vi "Untitled 4.vi"() -> ()   [LabVIEW 2011]
uses:
  emi Lib/System 01/0 - General/App/Loop control 2/Private/_emi_SMLoop Control Single.vi
  emi Lib/System 01/0 - General/S&E reporting/Private/_emi_ S&E Message type.ctl
  emi Lib/System 01/0 - General/S&E reporting/Private/_emi_ S&E Message.ctl
  <vilib>/Utility/file.llb/Write To Spreadsheet File (I64).vi
  emi Lib/System 01/0 - General/App/Loop control 2/Private/_emi_SMLoop Get State Single.vi
  Defenitions/LEIN Structure variations.ctl
  Defenitions/Error_system_def.ctl
  Defenitions/err/Controller error.ctl
  Defenitions/LEIN STAT 14 Debug system cluster.ctl
  Nodes/Controller local stat2.ctl
  Nodes/pressure stat2.ctl
  Nodes/solonoid stat2.ctl
  Tool/Stroker/Stat def/Stroker system stat2.ctl
  Defenitions/LEIN CMD List.ctl
  Defenitions/LEIN CMD Cluster.ctl
  Defenitions/LEIN cycle holder.ctl
  Defenitions/LEIN Reply Holder.ctl
  Defenitions/LEIN custom reply Q.ctl
  Nodes/tensionsub stat2.ctl
  Nodes/PSU stat2.ctl
  emi Lib/System 01/0 - General/App/Loop control/Private/_emi Loop status.ctl
  Defenitions/stat2/system status/Stat2 system task info.ctl
panel:
  out "Controller local.relay_status":u8 format="%.0b"
  out "controller task":T1
  out "pressure 2":bool
  out "Pressure 1":bool
  out "Solonoid":bool
  out "pressure 2":T2 {"sys register" format="%04x"}
  out "pressure 1":T2 {"sys register" format="%04x"}
  out "Solonoid":T1
  out "solonoid":T3 {"valve status" format="%02x"; "sys register" format="%04x"}
  out "Error":T4 {"system def error"."Module error mask" format="%08b"}
  out "Debug":T6
  out "ID":T7 {"LEIN implementation" format="%.0x"}
  out "Controler ID":u8[](array[numeric]) format="%.0x"
  out "Controler Debug":u8[](array[numeric]) format="%.0x"
  out "Controler error codes":u8[](array[numeric]) format="%.0x"
  in  "GetID Codes":bool
  in  "Get Debug codes":bool
  in  "Gett erro codes":bool
  out "DATA 3":u8[](array[numeric]) format="%.0x"
  in  "Array 2":u8[](array[numeric])=[1, 0, 1, 1, 2]
  in  "Solonoid":bool
  in  "Restart node":bool
  in  "TASK Data":u8[](array[numeric])=[120, 0, 50, 0, 0]
  in  "TASK ID":u8=49 format="%.0x"
  in  "TASK":bool
  in  "Reset err":bool
  out "DATA 2":u8[](array[numeric])=[240, 3, 105, 1, 0, 243, 11, 2, 32, 0, 6] format="%.0x"
  out "Reply":T8={"SID"=0, "ANF"=FALSE, "CMD"=enum."TASK", "DATA"=[]}
  in  "STAT ID":u8
  out "Numeric":i32
  out "PAss through answer":T8={"SID"=0, "ANF"=FALSE, "CMD"=enum."TASK", "DATA"=[]}
  out "SID 2":u8
  in  "Enable STAT2":bool=TRUE
  in  "Pass through":bool
  out "Boolean":bool
  in  "Ping":bool
  out "CMD":T8={"SID"=0, "ANF"=FALSE, "CMD"=enum."TASK", "DATA"=[]}
  in  "Stat":bool
  in  "Expected LEN":u16=60
  out "tid":u32
  out "PC-Control com errors":u32(graph)
  out "Node connected":u32(graph)
  out "Controller  current":u32(graph)
  out "Node  OSC":u32(graph)
  out "Node transducer":u32(graph)
  out "Node Temperature":u32(graph)
  out "Controller voltage":u32(graph)
  out "Accelerometer Ch 5":u32(graph)
  out "Accelerometer Ch 4":u32(graph)
  out "Accelerometer Ch 3":u32(graph)
  out "Accelerometer Ch 2":u32(graph)
  out "Accelerometer Ch 1":u32(graph)
  out "Accelerometer Ch 0":u32(graph)
  out "Sensor 2":u32(graph)
  out "Sensor 1":u32(graph)
  out "Temperature":u32(graph)
  out "Array":errorcluster[](array[cluster])
  in  "VISA com no":refnum<visa-resource-name>="COM 7"
  out "Loops":T10[](array[typedef])
  out "Received":i32
  out "Transmitt Qd":i32
  out "DATA":u8[](array[numeric]) format="%.0x"
  in  "SID":u8=42
  out "LEIN received":T8={"SID"=0, "ANF"=FALSE, "CMD"=enum."TASK", "DATA"=[]}
  # "In file: Tid, temperature, sensor 1,sensor 2,Acc 0, Acc1, Acc2, Acc3, Acc4, Acc5, Voltage, Current, Com errors, Node temperature, node transducerm, node osc, node discon (0 = connected)"
  # "OBS 1.2 diff OSCTUN location then 1.1"
  # "STAT DATA"
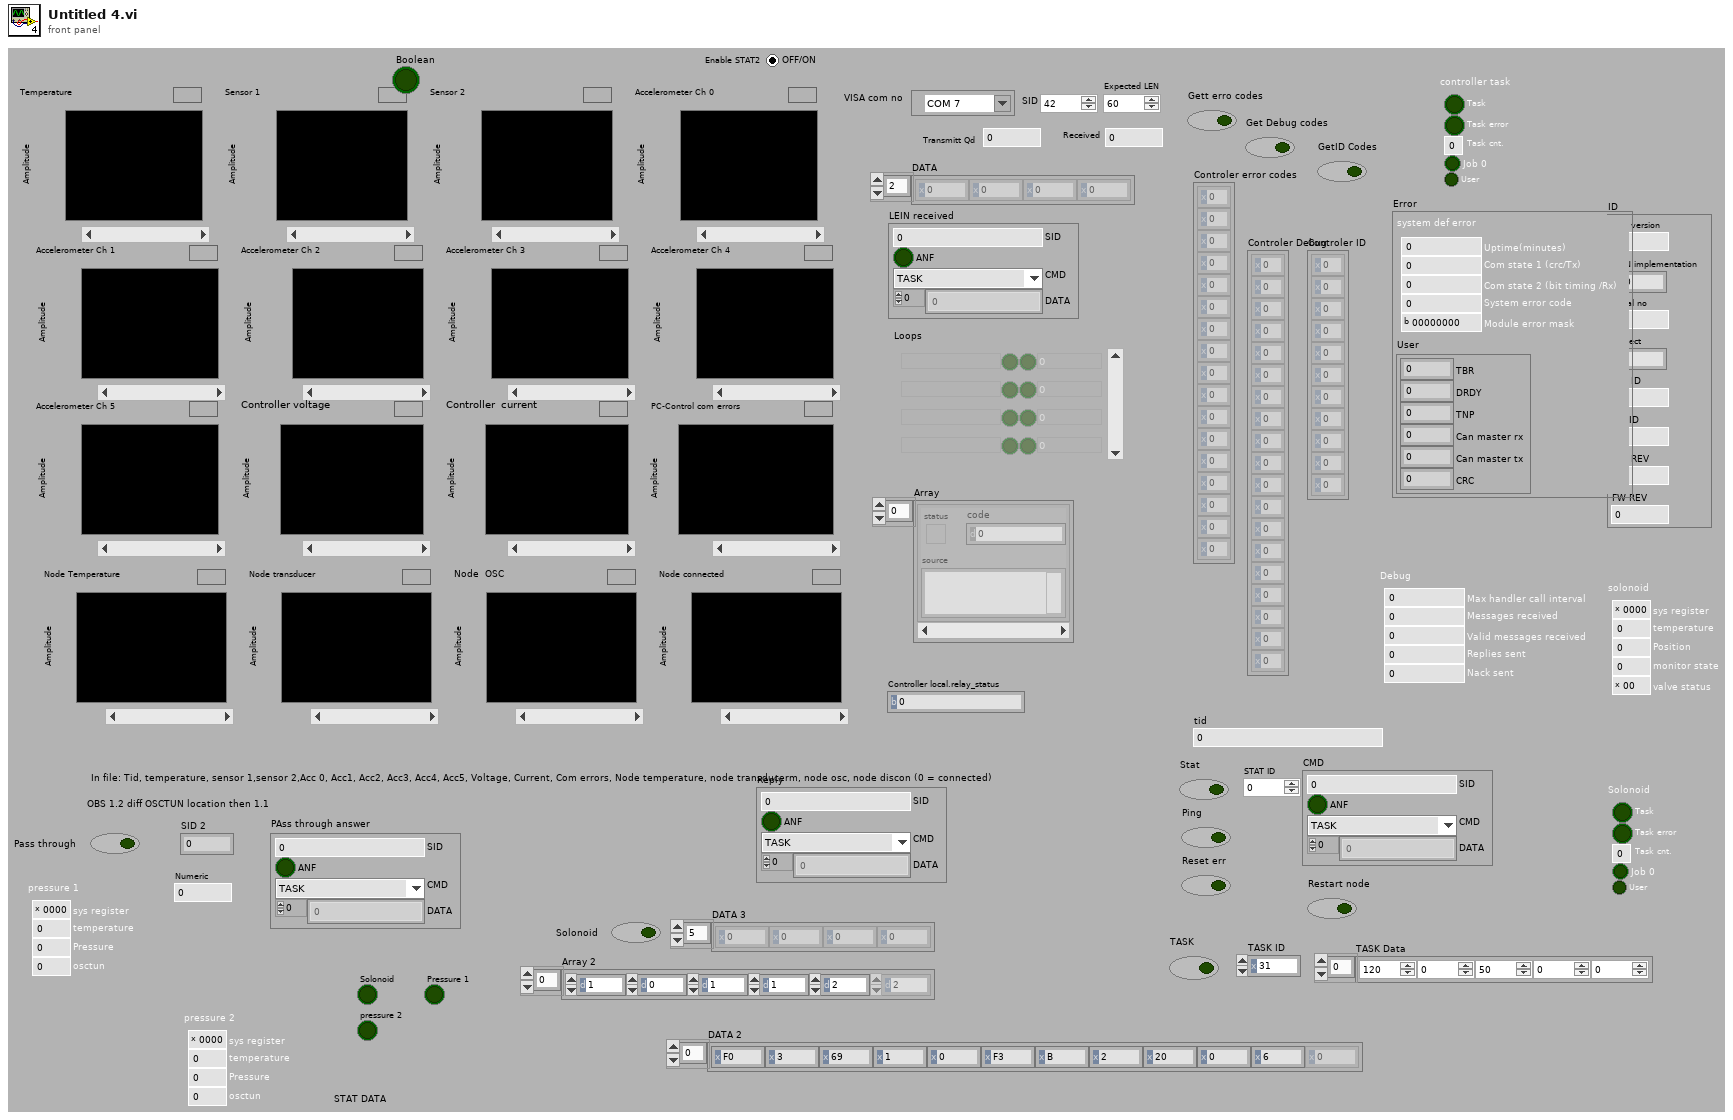
[diagram p1: front panel]
types:
  T1 = typedef "Stat2 system task info.ctl" = cluster{"Task":bool, "Task error":bool, "Task cnt.":u8, "Job 0":bool, "User":bool}
  T2 = typedef "pressure stat2.ctl" = cluster{"sys register":u16, "temperature":u16, "Pressure":u16, "osctun":u8}
  T3 = typedef "solonoid stat2.ctl" = cluster{"sys register":u16, "temperature":u16, "Position":i16, "monitor state":u8, "valve status":u8}
  T4 = typedef "Controller error.ctl" = cluster{"system def error":T5, "User":cluster{"TBR":u16, "DRDY":u16, "TNP":u16, "Can master rx":u8, "Can master tx":u8, "CRC":u16}}
  T5 = typedef "Error_system_def.ctl" = cluster{"Uptime(minutes)":u16, "Com state 1 (crc/Tx)":u8, "Com state 2 (bit timing /Rx)":u8, "System error code":u8, "Module error mask":u8}
  T6 = typedef "LEIN STAT 14 Debug system cluster.ctl" = cluster{"Max handler call interval":u16, "Messages received":u16, "Valid messages received":u16, "Replies sent":u16, "Nack sent":u16}
  T7 = cluster{"Lein version":u8, "LEIN implementation":u8, "Serial no":u16, "Project":u16, "HW ID":u8, "FW ID":u8, "HW REV":u8, "FW REV":u8}
  T8 = typedef "LEIN CMD Cluster.ctl" = cluster{"SID":u8, "ANF":bool, "CMD":T9, "DATA":u8[]}
  T9 = typedef "LEIN CMD List.ctl" = enum8{"ACTI", "TASK", "RES0", "STAT", "RES1", "RES2", "RES3", "USER"}
  T10 = typedef "_emi Loop status.ctl" = cluster{"Loop Name":string, "Enabled":bool, "Running":bool, "Restarts":i32}
  T11 = typedef "LEIN cycle holder.ctl" = cluster{"CMD":T8, "Retry if  unsucessful":bool, "LEIN reply holder":T12, "Reply in custom Q":bool, "LEIN custom reply Q":T13}
  T12 = typedef "LEIN Reply Holder.ctl" = cluster{"Reply msg(cmdif no reply)":T8, "Reply time":timestamp, "Valid reply":bool}
  T13 = typedef "LEIN custom reply Q.ctl" = refnum<queue>
  T14 = typedef "_emi_ S&E Message.ctl" = cluster{"Type":T15, "Originate time":dbl, "System":u8, "Loop":u16, "Sub ID":u16, "Elevated priority":bool, "E&S Message content":variant}
  T15 = typedef "_emi_ S&E Message type.ctl" = enum16{"Error/Warning", "Note", "Debug", "Event", "Alarm Analog", "Alarm Digital", "Annotation"}
  T16 = enum16{"big-endian, network order", "native, host order", "little-endian"}
  T17 = typedef "Stroker system stat2.ctl" = cluster{"Controller local":T18, "pressure 1":T2, "pressure 2":T2, "solonoid":T3, "PSU":T19, "Tension Sub 1":T20, "Tension Sub 2":T20}
  T18 = typedef "Controller local stat2.ctl" = cluster{"sys register":u16, "temperature":u16, "Input voltage":u16, "Input Current":u16, "Accelerometer ch0":u16, "Accelerometer ch1":u16, "Accelerometer ch2":u16, "Relay status":u8, "GPIO values":u8, "Sensor 1":i32, "Sensor 2":i32, "NA":u8, "High G monitoring":u8}
  T19 = typedef "PSU stat2.ctl" = cluster{"sys register":u16, "temperature":u16, "HV Voltage in":u16, "Main Voltage out":u16, "Main Current out":u16}
  T20 = typedef "tensionsub stat2.ctl" = cluster{"sys register":u16, "temperature":u16, "Tension":i16, "osctun":u8}
  T21 = typedef "LEIN Structure variations.ctl" = enum16{"LEIN08", "LEIN31", "LEIN63"}
  T22 = enum16{"open", "replace", "create", "open or create", "replace or create", "replace or create with confirmation"}
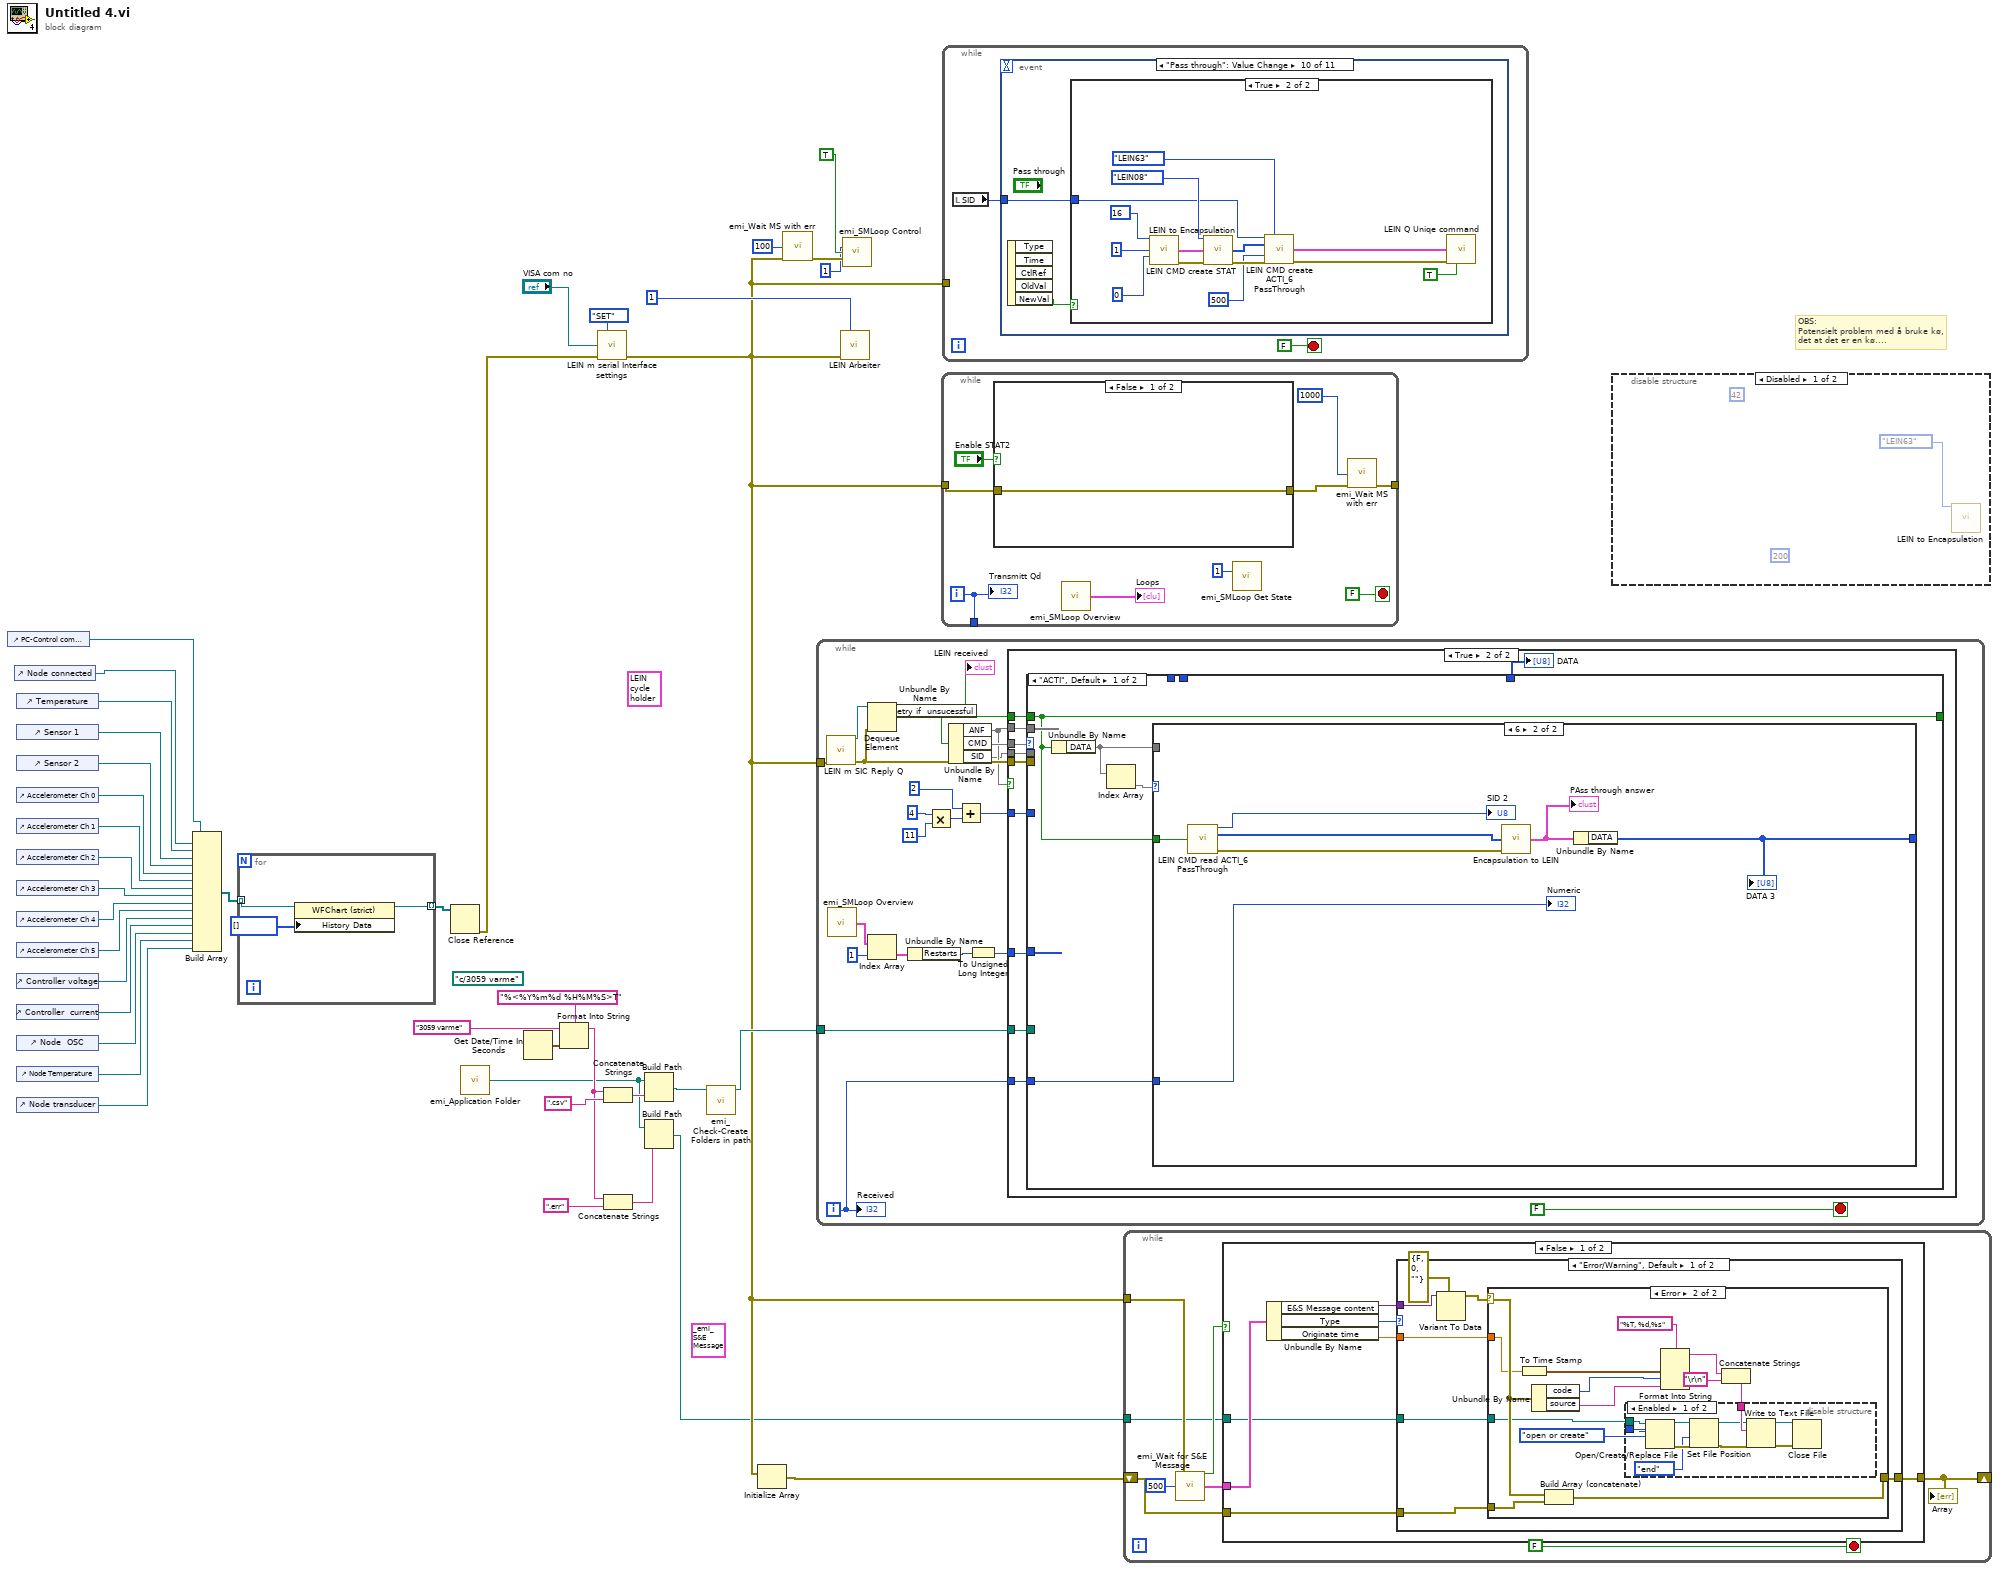
[diagram p0: block diagram]
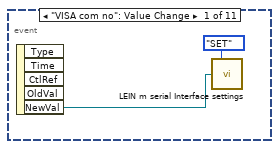
[diagram p3: hidden frame]
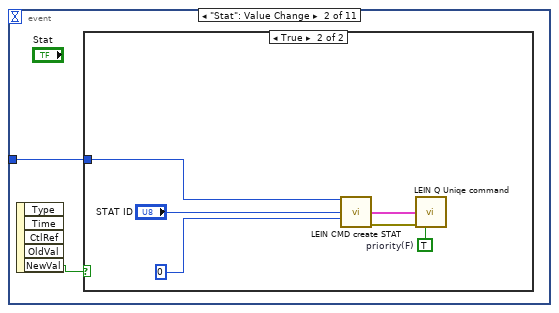
[diagram p4: hidden frame]
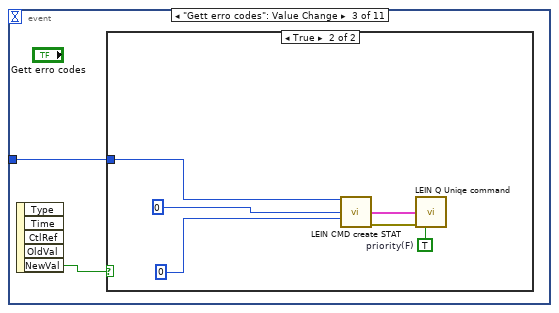
[diagram p6: hidden frame]
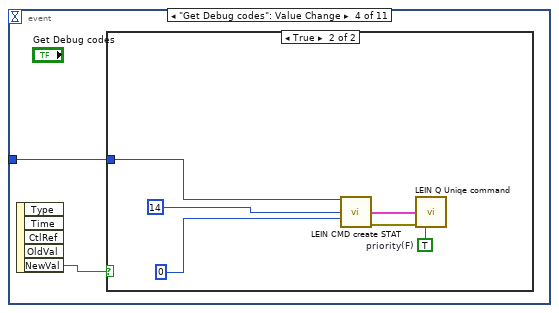
[diagram p8: hidden frame]
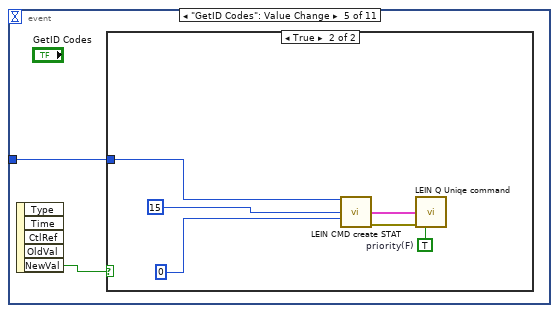
[diagram p10: hidden frame]
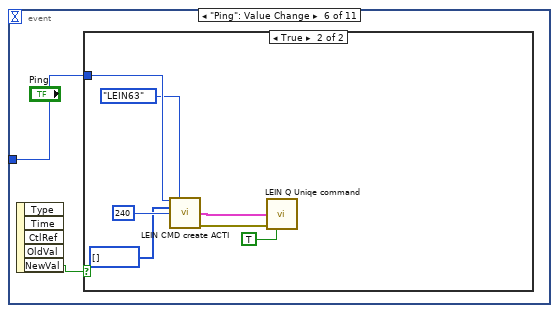
[diagram p12: hidden frame]
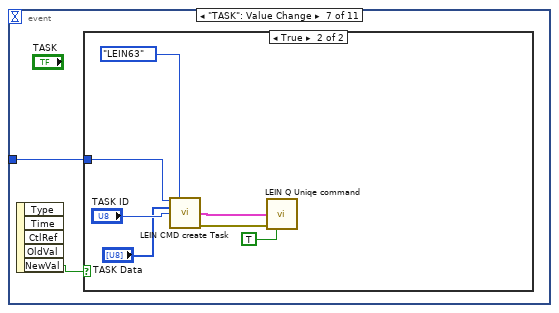
[diagram p14: hidden frame]
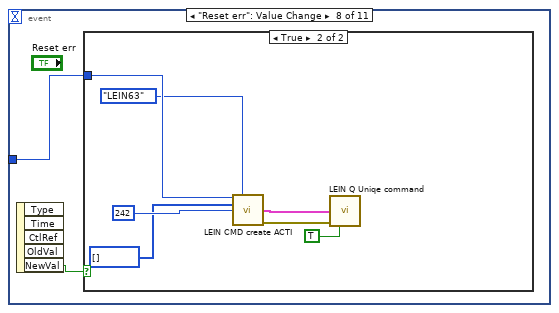
[diagram p16: hidden frame]
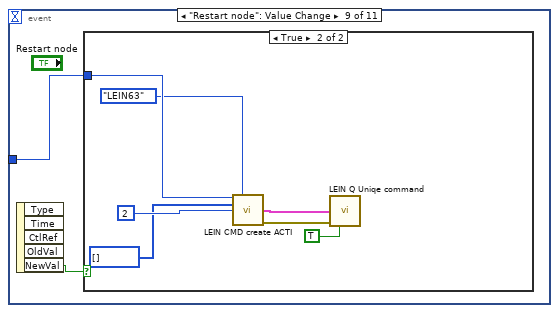
[diagram p18: hidden frame]
diagram:
  (unwired) T11 {"CMD"={"SID"=0, "ANF"=FALSE, "CMD"=enum."TASK", "DATA"=[]}, "Retry if  unsucessful"=FALSE, "LEIN reply holder"={"Reply msg(cmdif no reply)"={"SID"=0, "ANF"=FALSE, "CMD"=enum."ACTI", "DATA"=[]}, "Reply time"=timestamp(0 s since 1904-01-01), "Valid reply"=FALSE}, "Reply in custom Q"=FALSE, "LEIN custom reply Q"=refnum} ("element")
  (unwired) path "c:/3059 varme"
  (unwired) T14 {"Type"=enum."Error/Warning", "Originate time"=0.0, "System"=0, "Loop"=0, "Sub ID"=0, "Elevated priority"=FALSE, "E&S Message content"=variant} ("E&S Message")
  # "OBS:\nPotensielt problem med å bruke kø,\ndet at det er en kø...."
  n1 = control-ref of="PC-Control com errors"() -> (w9:refnum<vi>)
  n2 = control-ref of="Node connected"() -> (w10:refnum<vi>)
  n3 = control-ref of="Temperature"() -> (w27:refnum<vi>)
  n4 = control-ref of="Sensor 1"() -> (w26:refnum<vi>)
  n5 = control-ref of="Sensor 2"() -> (w25:refnum<vi>)
  n6 = control-ref of="Accelerometer Ch 0"() -> (w24:refnum<vi>)
  n7 = control-ref of="Accelerometer Ch 1"() -> (w23:refnum<vi>)
  n8 = control-ref of="Accelerometer Ch 2"() -> (w22:refnum<vi>)
  n9 = control-ref of="Accelerometer Ch 3"() -> (w21:refnum<vi>)
  n10 = control-ref of="Accelerometer Ch 4"() -> (w20:refnum<vi>)
  n11 = control-ref of="Accelerometer Ch 5"() -> (w19:refnum<vi>)
  n12 = control-ref of="Controller voltage"() -> (w18:refnum<vi>)
  n13 = control-ref of="Controller  current"() -> (w17:refnum<vi>)
  n14 = control-ref of="Node  OSC"() -> (w16:refnum<vi>)
  n15 = control-ref of="Node Temperature"() -> (w15:refnum<vi>)
  n16 = control-ref of="Node transducer"() -> (w14:refnum<vi>)
  n17 = Build Array(w9, w10, w27, w26, w25, w24, w23, w22, w21, w20, w19, w18, w17, w16, w15, w14) -> (w13:refnum<vi>[])
  n18 = for {
    tunnel: w13 -> [w43] mode=indexing
    tunnel: [w41] -> w12 mode=indexing
    n19 = property class="WFChart (strict)"(reference=w43, "History Data"=u32[] []) -> (reference out=w41:refnum<vi>)  [unwired: 1 in, 1 out]
  }
  n20 = Close Reference(reference=w12) -> (error out=w11:errorcluster)  [unwired: 1 in]
  n21 = call "emi_Application Folder.vi"() -> ("Dir"=w1:path)  [unwired: 14 in, 1 out]
  n22 = Get Date/Time In Seconds() -> (seconds since 1Jan1904=w32:timestamp)
  n23 = Format Into String(format string="%<%Y%m%d %H%M%S>T", initial string="3059 varme", w32) -> (resulting string=w4:string)  [unwired: 1 in, 1 out]
  n24 = call "LEIN m serial Interface settings.vi"("Action(GET)"=enum16{"GET", "SET"}."SET", "LEIN m serial VISA  name  in"="VISA com no", "error in (no error)"=w11) -> ("error out"=w8:errorcluster)  [unwired: 7 in, 5 out]
  n25 = Concatenate Strings(w4, ".csv" ("string")) -> (w7:string)
  n26 = Concatenate Strings(w4, ".err" ("string")) -> (w5:string)
  n27 = Build Path(base path=w1, name or relative path=w7) -> (appended path=w29:path)
  n28 = Build Path(base path=w1, name or relative path=w5) -> (appended path=w2:path)
  n29 = call "emi_Check-Create Folders in path.vi"("Path including file"=w29) -> ("Path out"=w28:path)  [unwired: 12 in, 2 out]
  n30 = Initialize Array(w8) -> (w33:errorcluster[])  [unwired: 1 in]
  n31 = call "emi_Wait MS with err.vi"("milliseconds to wait(0)"=u32 100 ("millisecond multiple(0)"), "error in (no error)"=w8) -> ("error out"=w36:errorcluster)  [unwired: 13 in]
  n32 = while {
    tunnel: w8 -> [w64]
    tunnel: w28 -> [w54]
    i -> [w44]
    stop <- FALSE stop-if-true
    n33 = call "LEIN m SIC Reply Q.vi"("error in (no error)"=w64) -> ("reply Q"=w62:refnum<queue>, "error out"=w60:errorcluster)  [unwired: 13 in]
    n34 = call "emi_SMLoop Overview.vi"() -> ("Loops"=w53:T10[])  [unwired: 14 in, 1 out]
    n35 = Dequeue Element(queue=w62, error in (no error)=w60) -> (element=w46:T11)  [unwired: 1 in, 3 out]
    n36 = Index Array(array=w53, index=1) -> (element=w51:T10)
    n37 = Unbundle By Name(w46) -> ("Retry if  unsucessful"=w45:bool)
    "LEIN received" <- w45
    n38 = Unbundle By Name(w51) -> ("Restarts"=w50:i32)
    n39 = Multiply(x=4 ("index"), y=11 ("index")) -> (x*y=w58:i32)
    n40 = Unbundle By Name(w45) -> ("ANF"=w48, "CMD"=w61, "SID"=w47)
    n41 = Add(x=2 ("index"), y=w58) -> (x+y=w55:i32)
    n42 = To Unsigned Long Integer(number=w50) -> (unsigned 32bit integer=w49:u32)
    n43 = case shown="True" w48 {
      tunnel: w61 -> [_ w74]
      tunnel: w45 -> [_ w73]
      tunnel: w60 -> [_ w72]
      tunnel: w55 -> [_ w70]
      tunnel: w54 -> [_ w69]
      tunnel: w49 -> [_ w68]
      tunnel: w48 -> [_ w67]
      tunnel: w47 -> [_ w66]
      tunnel: w44 -> [_ w65]
      frame False {
      }
      frame True {
        n44 = case shown="\"ACTI\", Default" w74 {
          tunnel: w73 -> [w76 w94]
          tunnel: w72 -> [_ w93]
          tunnel: [_ w91] -> w71
          tunnel: w70 -> [_ w92]
          tunnel: w69 -> [_ w90]
          tunnel: w68 -> [_ w89]
          tunnel: w67 -> [_ _]
          tunnel: [_ w88] -> _
          tunnel: [_ w87] -> _
          tunnel: w66 -> [_ w86]
          tunnel: [w76 _] -> _
          tunnel: w65 -> [w75 _]
          frame "ACTI", Default {
            n45 = Unbundle By Name(w76) -> ("DATA"=w77)
            n46 = Index Array(array=w77) -> (element=w78)  [unwired: 1 in]
            n47 = case shown="6" w78 {
              tunnel: w77 -> [_ _]
              tunnel: w76 -> [_ w83]
              tunnel: w75 -> [_ w81]
              tunnel: [_ w79] -> _
              frame 0, Default {
              }
              frame 6 {
                n48 = call "LEIN CMD read ACTI_6 PassThrough.vi"("CMD"=w83) -> ("SID"=→"SID 2":u8, "Reply from sub ID"=w84:u8[], "error out"=w85:errorcluster)  [unwired: 11 in, 1 out]
                n49 = call "Encapsulation to LEIN.vi"("Data and header"=w84, "error in (no error)"=w85) -> ("CMD out"=w80:T8)  [unwired: 10 in, 3 out]
                "PAss through answer" <- w80
                n50 = Unbundle By Name(w80) -> ("DATA"=w79:u8[])
                "DATA 3" <- w79
                "Numeric" <- w81
              }
            }
          }
          frame "STAT" {
            n51 = case shown="42" w86 {
              tunnel: w94 -> [w95 w96]
              tunnel: w93 -> [_ w103]
              tunnel: w92 -> [_ w98]
              tunnel: [_ w102] -> w91
              tunnel: w90 -> [_ w101]
              tunnel: w89 -> [_ w100]
              tunnel: [_ w99] -> w88
              tunnel: [_ w97] -> w87
              frame 0, Default {
                "CMD" <- w95
              }
              frame 42 {
                n52 = call "LEIN CMD read STAT.vi"("CMD"=w96, "error in (no error)"=w103) -> ("Data"=w102:u8[], "STAT ID"=w97:u8, "STAT Part"=w99:u8)  [unwired: 8 in, 3 out]
                n53 = case shown="0, Default" w97 {
                  selector: w97 -> [w104 _]
                  tunnel: w102 -> [w105 w183]
                  tunnel: w101 -> [_ w178]
                  tunnel: w100 -> [_ w172]
                  tunnel: w98 -> [_ _]
                  tunnel: [w107 _] -> _
                  tunnel: w96 -> [w107 _]
                  frame 0, Default {
                    n54 = case shown="0" w104 {
                      tunnel: w105 -> [_ w111 w116 w120]
                      frame 1, Default {
                      }
                      frame 0 {
                        n55 = Byte Array To String(unsigned byte array=w111) -> (string=w112:string)
                        n56 = Unflatten From String(type=T4 {"system def error"={"Uptime(minutes)"=0, "Com state 1 (crc/Tx)"=0, "Com state 2 (bit timing /Rx)"=0, "System error code"=0, "Module error mask"=0}, "User"={"TBR"=0, "DRDY"=0, "TNP"=0, "Can master rx"=0, "Can master tx"=0, "CRC"=0}} ("Cluster"), binary string=w112, data includes array or string size? (T)=FALSE, byte order (0:big-endian, network order)=T16."little-endian") -> (value=→"Error":T4)  [unwired: 1 in, 2 out]
                        "Controler error codes" <- w111
                      }
                      frame 14 {
                        n57 = Byte Array To String(unsigned byte array=w116) -> (string=w117:string)
                        n58 = Unflatten From String(type=T6 {"Max handler call interval"=0, "Messages received"=0, "Valid messages received"=0, "Replies sent"=0, "Nack sent"=0} ("Cluster 2"), binary string=w117, byte order (0:big-endian, network order)=T16."little-endian") -> (value=→"Debug":T6)  [unwired: 2 in, 2 out]
                        "Controler Debug" <- w116
                      }
                      frame 15 {
                        n59 = Byte Array To String(unsigned byte array=w120) -> (string=w119:string)
                        n60 = Unflatten From String(type=T7 {"Lein version"=0, "LEIN implementation"=0, "Serial no"=0, "Project"=0, "HW ID"=0, "FW ID"=0, "HW REV"=0, "FW REV"=0} ("Node ID"), binary string=w119, byte order (0:big-endian, network order)=T16."little-endian") -> (value=→"ID":T7)  [unwired: 2 in, 2 out]
                        "Controler ID" <- w120
                      }
                    }
                    n61 = Unbundle By Name(w107) -> ("DATA"=→"DATA 2")
                    "Reply" <- w107
                  }
                  frame 2 {
                    n62 = disable-structure shown="Disabled" {
                      frame Disabled {
                      }
                      frame Enabled {
                      }
                    }
                    n63 = Byte Array To String(unsigned byte array=w183) -> (string=w169:string)
                    n64 = Unflatten From String(type=T17 {"Controller local"={"sys register"=0, "temperature"=0, "Input voltage"=0, "Input Current"=0, "Accelerometer ch0"=0, "Accelerometer ch1"=0, "Accelerometer ch2"=0, "Relay status"=0, "GPIO values"=0, "Sensor 1"=0, "Sensor 2"=0, "NA"=0, "High G monitoring"=0}, "pressure 1"={"sys register"=0, "temperature"=0, "Pressure"=0, "osctun"=0}, "pressure 2"={"sys register"=0, "temperature"=0, "Pressure"=0, "osctun"=0}, "solonoid"={"sys register"=0, "temperature"=0, "Position"=0, "monitor state"=0, "valve status"=0}, "PSU"={"sys register"=0, "temperature"=0, "HV Voltage in"=0, "Main Voltage out"=0, "Main Current out"=0}, "Tension Sub 1"={"sys register"=0, "temperature"=0, "Tension"=0, "osctun"=0}, "Tension Sub 2"={"sys register"=0, "temperature"=0, "Tension"=0, "osctun"=0}} ("system stat2"), binary string=w169, byte order (0:big-endian, network order)=T16."little-endian") -> (value=w167:T17)  [unwired: 2 in, 2 out]
                    n65 = Unbundle By Name(w167) -> ("Controller local.sys register"=w126:u16, "pressure 1.osctun"=w153:u8, "pressure 1.Pressure"=w154:u16, "pressure 1.temperature"=w155:u16, "pressure 1.sys register"=w152:u16, "Controller local.temperature"=w166:u16, "sensor 1"=w165:i32, "sensor 2"=w164:i32, "Controller local.Accelerometer ch0"=w163:u16, "Controller local.Accelerometer ch1"=w162:u16, "Controller local.Accelerometer ch2"=w161:u16, "Accelerometer ch3 (hi-g)"=w160:u16, "Accelerometer ch4 (hi-g)"=w159:u16, "Accelerometer ch5 (hi-g)"=w158:u16, "Controller local.Input voltage"=w157:u16, "Controller local.Input Current"=w156:u16, "solonoid"=→"solonoid":T3, "solonoid.sys register"=w147:u16, "pressure 1"=→"pressure 1":T2, "pressure 2"=→"pressure 2":T2, "pressure 1.sys register"=w130:u16, "pressure 2.sys register"=w128:u16, "relay_status"=→"Controller local.relay_status":u8)
                    n66 = call "Lein stat2 read system status.vi"("sys register"=w128) -> ("Connected"=→"pressure 2":bool)  [unwired: 7 in, 7 out]
                    n67 = call "Lein stat2 read system status.vi"("sys register"=w130) -> ("Connected"=→"Pressure 1":bool)  [unwired: 7 in, 7 out]
                    n68 = call "Lein stat2 read system status.vi"("sys register"=w147) -> ("Connected"=→"Solonoid":bool, "Task"=→"Solonoid":T1)  [unwired: 7 in, 6 out]
                    n69 = call "Lein stat2 read system status.vi"("sys register"=w152) -> ("Connected"=w151:bool)  [unwired: 7 in, 7 out]
                    n70 = To Unsigned Long Integer(number=w156) -> (unsigned 32bit integer=w135:u32)
                    "Controller  current" <- w135
                    n71 = To Unsigned Long Integer(number=w157) -> (unsigned 32bit integer=w136:u32)
                    "Controller voltage" <- w136
                    n72 = To Unsigned Long Integer(number=w166) -> (unsigned 32bit integer=w145:u32)
                    "Temperature" <- w145
                    n73 = To Unsigned Long Integer(number=w159) -> (unsigned 32bit integer=w138:u32)
                    "Accelerometer Ch 4" <- w138
                    n74 = To Unsigned Long Integer(number=w158) -> (unsigned 32bit integer=w137:u32)
                    "Accelerometer Ch 5" <- w137
                    n75 = To Unsigned Long Integer(number=w162) -> (unsigned 32bit integer=w141:u32)
                    "Accelerometer Ch 1" <- w141
                    n76 = To Unsigned Long Integer(number=w163) -> (unsigned 32bit integer=w142:u32)
                    "Accelerometer Ch 0" <- w142
                    n77 = To Unsigned Long Integer(number=w160) -> (unsigned 32bit integer=w139:u32)
                    "Accelerometer Ch 3" <- w139
                    n78 = To Unsigned Long Integer(number=w165) -> (unsigned 32bit integer=w144:u32)
                    "Sensor 1" <- w144
                    n79 = To Unsigned Long Integer(number=w164) -> (unsigned 32bit integer=w143:u32)
                    "Sensor 2" <- w143
                    n80 = Boolean To (0,1)(Boolean=w151) -> (0, 1=w150:i16)
                    n81 = To Unsigned Long Integer(number=w161) -> (unsigned 32bit integer=w140:u32)
                    "Accelerometer Ch 2" <- w140
                    n82 = To Unsigned Long Integer(number=w150) -> (unsigned 32bit integer=w149:u32)
                    n83 = Get Date/Time In Seconds() -> (seconds since 1Jan1904=w174:timestamp)
                    n84 = To Unsigned Long Integer(number=w149) -> (unsigned 32bit integer=→"Node connected":u32)
                    n85 = To Unsigned Long Integer(number=w174) -> (unsigned 32bit integer=w173:u32)
                    "tid" <- w173
                    n86 = To Unsigned Long Integer(number=w155) -> (unsigned 32bit integer=→"Node Temperature":u32)
                    n87 = To Unsigned Long Integer(number=w154) -> (unsigned 32bit integer=→"Node transducer":u32)
                    n88 = To Unsigned Long Integer(number=w153) -> (unsigned 32bit integer=→"Node  OSC":u32)
                    n89 = Build Array(w173, w145, w144, w143, w142, w141, w140, w139, w138, w137, w136, w135, w172, w155, w154, w153, w149) -> (w179:u32[])
                    n90 = call "Lein stat2 read system status.vi"("sys register"=w126) -> ("Task"=→"controller task":T1)  [unwired: 7 in, 7 out]
                    n91 = call-poly <vilib>:"Write To Spreadsheet File.vi"("delimiter (\\t)"="," ("delimiter (\\t)"), "append to file? (new file:F)"=TRUE, "1D data"=w179, "file path (dialog if empty)"=w178) -> ()  [unwired: 4 in, 1 out]
                    n92 = feedback #1() -> (w171:bool)  [unwired: 1 in]
                    n93 = Not(x=w171) -> (.not. x?=w170:bool)
                    "Boolean" <- w170
                    n94 = feedback-in #1(w170) -> ()
                    "PC-Control com errors" <- w172
                  }
                }
              }
            }
          }
        }
        "DATA" <- w71
      }
    }
    "Received" <- w44
  }
  n95 = call "LEIN Arbeiter.vi"("LEIN m Serial Transmitt Loop ID"=1, "error Inn"=w8) -> ()  [unwired: 14 in]
  n96 = call-poly "emi_SMLoop Control.vi"("Loop ID in"=u16 1, "Enable"=TRUE, "error in (no error)"=w36) -> ()  [unwired: 11 in, 2 out]
  n97 = while {
    tunnel: w8 -> [w185]
    tunnel: [w191] -> _
    tunnel: [w190] -> _
    i -> [w191]
    stop <- FALSE stop-if-true
    n98 = case shown="False" "Enable STAT2" {
      tunnel: [w193 w201] -> w186
      tunnel: w185 -> [w193 w199]
      frame False {
      }
      frame True {
        n99 = call "LEIN CMD read STATs by len.vi"("SID"="SID", "LEIN Variation"=LEIN_Structure_variations."LEIN63", "Expected LEN"="Expected LEN", "STAT ID"=u8 2, "error in"=w199) -> ("STATs"=w197:T8[], "error out"=w198:errorcluster)  [unwired: 9 in]
        n100 = for {
          N -> [w202]
          tunnel: [w206] -> w201
          tunnel: w198 -> [w205]
          tunnel: w197 -> [w204] mode=indexing
          tunnel: [w203] -> _ mode=indexing
          tunnel: [w202] -> _ mode=indexing
          i -> [w203]
          n101 = call "LEIN Q Uniqe command.vi"("CMD"=w204, "error in"=w205) -> ("error out"=w206:errorcluster)  [unwired: 13 in]
        }
      }
    }
    n102 = call "emi_SMLoop Overview.vi"() -> ("Loops"=→"Loops":T10[])  [unwired: 14 in, 1 out]
    n103 = call-poly "emi_SMLoop Get State.vi"("Loop ID in"=u16 1) -> ()  [unwired: 8 in, 7 out]
    n104 = call "emi_Wait MS with err.vi"("milliseconds to wait(0)"=u32 1000 ("millisecond multiple(0)"), "error in (no error)"=w186) -> ("error out"=w190:errorcluster)  [unwired: 13 in]
    "Transmitt Qd" <- w191
  }
  n105 = while {
    tunnel: w8 -> [_]
    stop <- FALSE stop-if-true
    n106 = local read "SID"() -> (w207:u8)
    n107 = event shown="[9] \"Pass through\": Value Change" {
      selector: _ -> [_ _ _ _ _ _ _ _ _ _ _]
      dyn-events: _ -> [_ _ _ _ _ _ _ _ _ _ _]
      timeout: _ -> [_ _ _ _ _ _ _ _ _ _ _]
      tunnel: w207 -> [_ w211 w219 w227 w235 w243 w252 w261 w270 w279 w295]
      event "VISA com no": Value Change {
        n108 = event-data() -> ("NewVal"=w209:refnum<visa-resource-name>)  [unwired: 1 in, 4 out]
        n109 = call "LEIN m serial Interface settings.vi"("Action(GET)"=enum16{"GET", "SET"}."SET", "LEIN m serial VISA  name  in"=w209) -> ()  [unwired: 8 in, 6 out]
      }
      event "Stat": Value Change {
        n110 = event-data() -> ("NewVal"=w212:bool)  [unwired: 1 in, 4 out]
        n111 = case shown="True" w212 {
          tunnel: w211 -> [_ w216]
          frame False {
          }
          frame True {
            w215 = TRUE  # priority(F)
            n112 = call "LEIN CMD create STAT.vi"("SID"=w216, "STAT ID"="STAT ID", "STAT Part"=u8 0) -> ("CMD"=w217:T8, "error out"=w218:errorcluster)  [unwired: 11 in]
            n113 = call "LEIN Q Uniqe command.vi"("CMD"=w217, "error in"=w218, "priority(F)"=w215) -> ()  [unwired: 12 in, 1 out]
          }
        }
      }
      event "Gett erro codes": Value Change {
        n114 = event-data() -> ("NewVal"=w220:bool)  [unwired: 1 in, 4 out]
        n115 = case shown="True" w220 {
          tunnel: w219 -> [_ w224]
          frame False {
          }
          frame True {
            w223 = TRUE  # priority(F)
            n116 = call "LEIN CMD create STAT.vi"("SID"=w224, "STAT ID"=u8 0, "STAT Part"=u8 0) -> ("CMD"=w225:T8, "error out"=w226:errorcluster)  [unwired: 11 in]
            n117 = call "LEIN Q Uniqe command.vi"("CMD"=w225, "error in"=w226, "priority(F)"=w223) -> ()  [unwired: 12 in, 1 out]
          }
        }
      }
      event "Get Debug codes": Value Change {
        n118 = event-data() -> ("NewVal"=w228:bool)  [unwired: 1 in, 4 out]
        n119 = case shown="True" w228 {
          tunnel: w227 -> [_ w232]
          frame False {
          }
          frame True {
            w231 = TRUE  # priority(F)
            n120 = call "LEIN CMD create STAT.vi"("SID"=w232, "STAT ID"=u8 14, "STAT Part"=u8 0) -> ("CMD"=w233:T8, "error out"=w234:errorcluster)  [unwired: 11 in]
            n121 = call "LEIN Q Uniqe command.vi"("CMD"=w233, "error in"=w234, "priority(F)"=w231) -> ()  [unwired: 12 in, 1 out]
          }
        }
      }
      event "GetID Codes": Value Change {
        n122 = event-data() -> ("NewVal"=w236:bool)  [unwired: 1 in, 4 out]
        n123 = case shown="True" w236 {
          tunnel: w235 -> [_ w240]
          frame False {
          }
          frame True {
            w239 = TRUE  # priority(F)
            n124 = call "LEIN CMD create STAT.vi"("SID"=w240, "STAT ID"=u8 15, "STAT Part"=u8 0) -> ("CMD"=w241:T8, "error out"=w242:errorcluster)  [unwired: 11 in]
            n125 = call "LEIN Q Uniqe command.vi"("CMD"=w241, "error in"=w242, "priority(F)"=w239) -> ()  [unwired: 12 in, 1 out]
          }
        }
      }
      event "Ping": Value Change {
        n126 = event-data() -> ("NewVal"=w244:bool)  [unwired: 1 in, 4 out]
        n127 = case shown="True" w244 {
          tunnel: w243 -> [_ w250]
          frame False {
          }
          frame True {
            n128 = call "LEIN CMD create ACTI.vi"("SID"=w250, "LEIN Variation"=LEIN_Structure_variations."LEIN63", "Data"=u8[] [], "ACTI ID"=u8 240) -> ("CMD"=w249:T8, "error out"=w251:errorcluster)  [unwired: 10 in]
            n129 = call "LEIN Q Uniqe command.vi"("CMD"=w249, "error in"=w251, "priority(F)"=TRUE) -> ()  [unwired: 12 in, 1 out]
          }
        }
      }
      event "TASK": Value Change {
        n130 = event-data() -> ("NewVal"=w253:bool)  [unwired: 1 in, 4 out]
        n131 = case shown="True" w253 {
          tunnel: w252 -> [_ w259]
          frame False {
          }
          frame True {
            n132 = call "LEIN CMD create Task.vi"("SID"=w259, "LEIN Variation"=LEIN_Structure_variations."LEIN63", "Data"="TASK Data", "TASK ID"="TASK ID") -> ("CMD"=w258:T8, "error out"=w260:errorcluster)  [unwired: 10 in]
            n133 = call "LEIN Q Uniqe command.vi"("CMD"=w258, "error in"=w260, "priority(F)"=TRUE) -> ()  [unwired: 12 in, 1 out]
          }
        }
      }
      event "Reset err": Value Change {
        n134 = event-data() -> ("NewVal"=w262:bool)  [unwired: 1 in, 4 out]
        n135 = case shown="True" w262 {
          tunnel: w261 -> [_ w268]
          frame False {
          }
          frame True {
            n136 = call "LEIN CMD create ACTI.vi"("SID"=w268, "LEIN Variation"=LEIN_Structure_variations."LEIN63", "Data"=u8[] [], "ACTI ID"=u8 242) -> ("CMD"=w267:T8, "error out"=w269:errorcluster)  [unwired: 10 in]
            n137 = call "LEIN Q Uniqe command.vi"("CMD"=w267, "error in"=w269, "priority(F)"=TRUE) -> ()  [unwired: 12 in, 1 out]
          }
        }
      }
      event "Restart node": Value Change {
        n138 = event-data() -> ("NewVal"=w271:bool)  [unwired: 1 in, 4 out]
        n139 = case shown="True" w271 {
          tunnel: w270 -> [_ w277]
          frame False {
          }
          frame True {
            n140 = call "LEIN CMD create ACTI.vi"("SID"=w277, "LEIN Variation"=LEIN_Structure_variations."LEIN63", "Data"=u8[] [], "ACTI ID"=u8 2) -> ("CMD"=w276:T8, "error out"=w278:errorcluster)  [unwired: 10 in]
            n141 = call "LEIN Q Uniqe command.vi"("CMD"=w276, "error in"=w278, "priority(F)"=TRUE) -> ()  [unwired: 12 in, 1 out]
          }
        }
      }
      event "Pass through": Value Change {
        n142 = event-data() -> ("NewVal"=w280:bool)  [unwired: 1 in, 4 out]
        n143 = case shown="True" w280 {
          tunnel: w279 -> [_ w287]
          frame False {
          }
          frame True {
            n144 = call "LEIN CMD create STAT.vi"("SID"=u8 16, "STAT ID"=u8 1, "STAT Part"=u8 0 ("STAT ID")) -> ("CMD"=w288:T8, "error out"=w289:errorcluster)  [unwired: 11 in]
            n145 = call "LEIN to Encapsulation.vi"("LEIN Variation"=LEIN_Structure_variations."LEIN08", "CMD"=w288, "error in (no error)"=w289) -> ("Data and header"=w284:u8[], "error out"=w285:errorcluster)  [unwired: 8 in, 3 out]
            n146 = call "LEIN CMD create ACTI_6 PassThrough.vi"("SID"=w287, "LEIN Variation"=LEIN_Structure_variations."LEIN63", "LEIN ecapsulated data (header and data)"=w284, "Sub Timeout (ms)"=u16 500, "error in (no error)"=w285) -> ("CMD"=w283:T8, "error out"=w282:errorcluster)  [unwired: 9 in]
            n147 = call "LEIN Q Uniqe command.vi"("CMD"=w283, "error in"=w282, "priority(F)"=TRUE) -> ()  [unwired: 12 in, 1 out]
          }
        }
      }
      event "Solonoid": Value Change {
        n148 = event-data() -> ("NewVal"=w296:bool)  [unwired: 1 in, 4 out]
        n149 = case shown="True" w296 {
          tunnel: w295 -> [_ w309]
          frame False {
          }
          frame True {
            w297 = LEIN_Structure_variations."LEIN08" ("LEIN Variation")
            n150 = call "LEIN CMD create Task.vi"("SID"=u8 16, "LEIN Variation"=w297, "Data"="Array 2", "TASK ID"=u8 50 ("STAT ID")) -> ("CMD"=w301:T8, "error out"=w302:errorcluster)  [unwired: 10 in]
            n151 = call "LEIN to Encapsulation.vi"("LEIN Variation"=w297, "CMD"=w301, "error in (no error)"=w302) -> ("Data and header"=w306:u8[], "error out"=w307:errorcluster)  [unwired: 8 in, 3 out]
            n152 = call "LEIN CMD create ACTI_6 PassThrough.vi"("SID"=w309, "LEIN Variation"=LEIN_Structure_variations."LEIN63", "LEIN ecapsulated data (header and data)"=w306, "Sub Timeout (ms)"=u16 100, "error in (no error)"=w307) -> ("CMD"=w305:T8, "error out"=w304:errorcluster)  [unwired: 9 in]
            n153 = call "LEIN Q Uniqe command.vi"("CMD"=w305, "error in"=w304, "priority(F)"=TRUE) -> ()  [unwired: 12 in, 1 out]
          }
        }
      }
    }
  }
  n154 = while {
    tunnel: w8 -> [w318]
    shift-right: [w315] -> _
    shift-left: w33 -> [w314]
    tunnel: w2 -> [w311]
    stop <- FALSE stop-if-true
    n155 = call "emi_Wait for S&E Message.vi"("timeout in ms (5)"=500, "error in (no error)"=w318) -> ("timed out?"=w313:bool, "E&S Message"=w316:T14)  [unwired: 11 in, 1 out]
    n156 = case shown="False" w313 {
      tunnel: w316 -> [w324 _]
      tunnel: [w323 w358] -> w315
      tunnel: w314 -> [w322 w358]
      tunnel: w311 -> [w319 _]
      frame False {
        n157 = Unbundle By Name(w324) -> ("E&S Message content"=w321:variant, "Type"=w325:T15, "Originate time"=w320:dbl)
        n158 = case shown="\"Error/Warning\", Default" w325 {
          tunnel: [w332 w357] -> w323
          tunnel: w322 -> [w331 w357]
          tunnel: w321 -> [w330 _]
          tunnel: w320 -> [w327 _]
          tunnel: w319 -> [w326 _]
          frame "Error/Warning", Default {
            n159 = Variant To Data(type=errorcluster {"status"=FALSE, "code"=0, "source"=""} ("error out"), Variant=w330) -> (data=w328:errorcluster)  [unwired: 1 in, 1 out]
            n160 = case shown="Error" w328 {
              selector: w328 -> [_ w344]
              tunnel: [w333 w346] -> w332
              tunnel: w331 -> [w333 w345]
              tunnel: w327 -> [_ w341]
              tunnel: w326 -> [_ w334]
              frame No Error {
              }
              frame Error {
                n161 = To Time Stamp(1:w341) -> (0:w340:timestamp)
                n162 = Unbundle By Name(w344) -> ("code"=w343:i32, "source"=w342:string)
                n163 = Build Array (concatenate)(w344, w345) -> (w346:errorcluster[])
                n164 = Format Into String(format string="%T, %d,%s", w340, w343, w342) -> (resulting string=w338:string)  [unwired: 2 in, 1 out]
                n165 = Concatenate Strings(w338, "\r\n") -> (w336:string)
                n166 = disable-structure shown="Enabled" {
                  disable-tunnel: w336 -> [w353 _]
                  disable-tunnel: T22."open or create" ("operation (0:open)") -> [w352 _]
                  disable-tunnel: w334 -> [w351 _]
                  frame Enabled {
                    n167 = Open/Create/Replace File(file path (use dialog)=w351, operation (0:open)=w352) -> (refnum out=w354:refnum<file>, error out=w349:errorcluster)  [unwired: 4 in, 1 out]
                    n168 = Set File Position(refnum=w354, from (0:start)=enum16{"start", "end", "current"}."end", error in=w349) -> (refnum out=w350:refnum<file>, error out=w348:errorcluster)  [unwired: 1 in]
                    n169 = Write to Text File(file (use dialog)=w350, text=w353, error in=w348) -> (refnum out=w355:refnum<file>, error out=w356:errorcluster)  [unwired: 1 in, 1 out]
                    n170 = Close File(refnum=w355, error in=w356) -> ()  [unwired: 2 out]
                  }
                  frame Disabled {
                  }
                }
              }
            }
          }
          frame "Note" {
          }
        }
      }
      frame True {
      }
    }
    "Array" <- w315
  }
  n171 = disable-structure shown="Disabled" {
    frame Disabled {
      w362 = u16 200 ("Sub Timeout (ms)")
      w363 = u8 42 ("SID")
      n172 = call "LEIN to Encapsulation.vi"("LEIN Variation"=LEIN_Structure_variations."LEIN63") -> ("CMD"=w359:T8, "error in (no error)"=w361:errorcluster)  [unwired: 8 in, 5 out]
    }
    frame Enabled {
    }
  }
